vi "FactorPass.vi"(7 "Robot":dbl[](array[numeric]), 8 "error in (no error)":errorcluster, 9 "OffensivePlay":T1=enum."TableWithStriker", 10 "Game":refnum<class "Game.lvclass">, 11 "Utilities in":refnum<class "Utilities.lvclass">) -> (0 "error out":errorcluster, 2 "Critério de marcação Normalizado":dbl, 3 "Utilities out":refnum<class "Utilities.lvclass">)   [LabVIEW 2023, in "Utilities.lvclass"]
uses:
  Utilities.lvclass
  Game_class/Game.lvclass
  Team_class/OffensivePlay.ctl
  Robot_class/roles.ctl
  Game_class/Game.lvclass/Game.ctl
  Object_class/Object.lvclass/Object.ctl
  Referee_class/Referee.lvclass/Referee.ctl
  Team_class/Team.lvclass/Team.ctl
  Robot_class/Robot.lvclass/Robot.ctl
  <vilib>/Analysis/_algsub.llb/Real Vector Norm.vi
  Object_class/Read x.vi
  Object_class/Read y.vi
  Robot_class/Read id.vi
  40316e39-9fcb-4662-8d02-ffa9e406c10e.vi
  Game_class/Read BallRef.vi
  Game_class/Read Referee.vi
  Game_class/Read FieldRef.vi
  Game_class/Read EnemyRef.vi
  Game_class/Read Utilities.lvclass.vi
  Game_class/Read OffensiveTeam.vi
  Team_class/Read RobotRef.vi
  Referee_class/Read enemy_goalie_id.vi
  <vilib>/Array/Sort 2D Array - Pop Stack.vi
  <vilib>/Array/Sort 2D Array - Push Stack.vi
  40316e39-9fcb-4662-8d02-ffa9e406c10e.vi/269d4b3b-47f5-49e3-8884-44851e4dd9d5.vi
  40316e39-9fcb-4662-8d02-ffa9e406c10e.vi/6d99389c-673d-4efb-bf33-19b32bcf4cf8.vi
  Ally_class/Ally.lvclass
  C:/Users/ebert/Documents/codes/SSL/repo/SSL_AI/Team_class/Team.lvclass
  Robot_class/Robot.lvclass
  C:/Users/ebert/Documents/codes/SSL/repo/SSL_AI/Object_class/Object.lvclass
  Enemy_class/Enemy.lvclass
  Ball_class/Ball.lvclass
  Referee_class/Referee.lvclass
  Field_class/Field.lvclass
  <vilib>/Analysis/NI_AALPro.lvlib
panel:
  out "t":dbl
  out "id inimigo \nmaior diferença \nde tempo":dbl
  out "Array out":dbl[][](array[numeric])
  out "Dif. tempo\ninimigo bola":dbl
  out "menor dist":dbl
  out "Robô marcado?":bool=TRUE
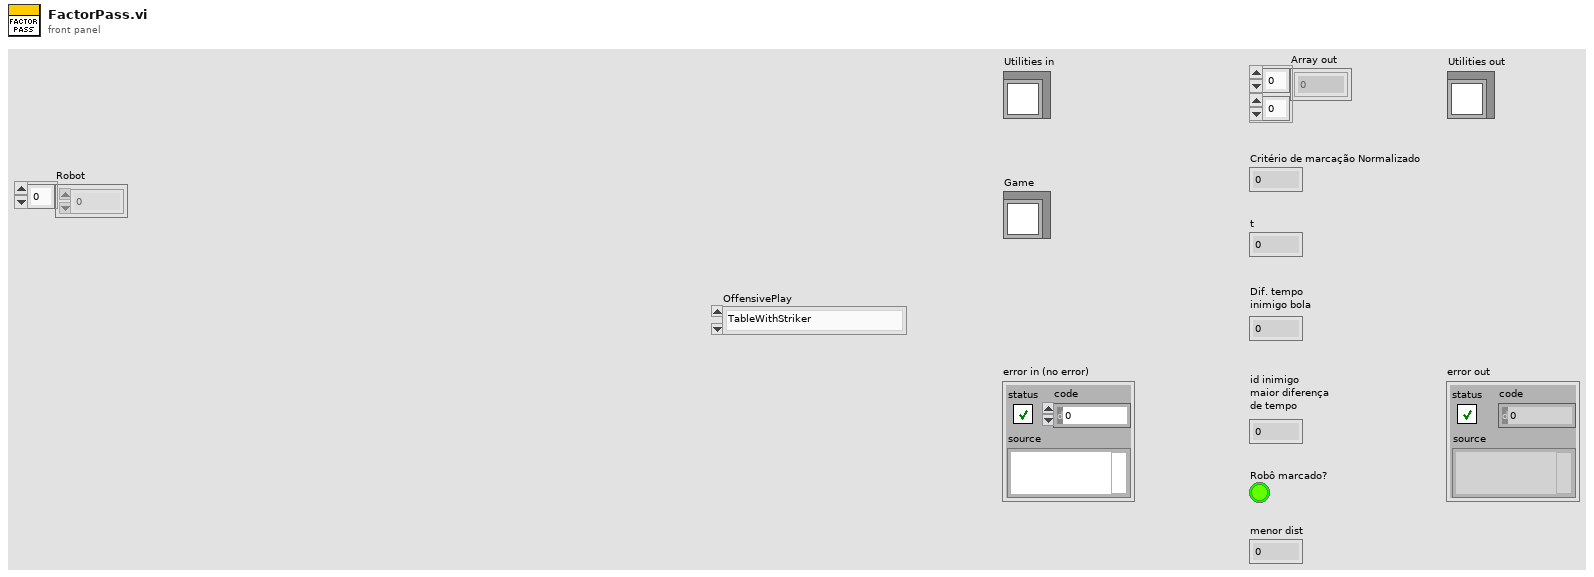
[diagram p1: front panel]
types:
  T1 = typedef "OffensivePlay.ctl" = enum16{"5RobotsPassGamePlay", "5PreparePassGame", "5RobotsKeeperGame", "KeeperPassToStriker", "5RobotsNormalGamePlay", "PrepareKeeperPass", "ACBPass", "ABCPass", "PrepareTriplePass", "TableWithStriker", "TableWith2ndStrikerPlay", "PrepareDoublePass", "PrepareRollToPass", "SimplePass", "PreparePass", "PassToStriker", "BallOutOfField", "PassTo2ndStriker", "StopOffensive", "Prepare Penalty Enemy", "EnemyPossessionAtEnemyField", "EnemyPossesionAtOurField", "TestPlay", "PreparePenaltyAlly", "KickPenaltyAlly", "PrepareKickoffAlly", "PrepareKickoffEnemy", "IndirectEnemy", "DirectEnemy", "PreparePassInGame1", "NormalGame", "DirectKick", "Pass", "Halt", "Timeout", "PassPlay", "PenaltyEnemy"}
  T2 = typedef "roles.ctl" = enum16{"SimpleBallPlacement", "BallPlacementAllyPasser", "BallPlacementAllyReceiver", "BallPlacementEnemy", "5Robots5th", "PassBestReceiver", "5Robots4th", "5Robots3rd", "5Robots2nd", "5Robots1st", "PassBestRobot", "WaitPass", "ABCThirdKicker", "ABCFirstKicker", "ABCSecondKicker", "Tabler", "TableFinalizer", "PrepareRollToPassRoller", "PrepareRollToPassReceiver", "SimplePassRoll", "SimplePassRollReceiver", "PenaltyDefense", "PreparePassReceiver 2", "PreparePassReceiver 1", "PassObserver", "Timeout", "Goto", "ZigZag", "None", "BallOutOfField", "DefenderArea", "Duelist", "AttackerStop", "FollowAttacker", "KeeperRole", "KickPenalty", "AttackerAimGoal", "AttackerBlock", "Marker", "Halt", "Shoot", "PassKicker", "PassReceiver", "TestRole", "PenaltyAttacker"}
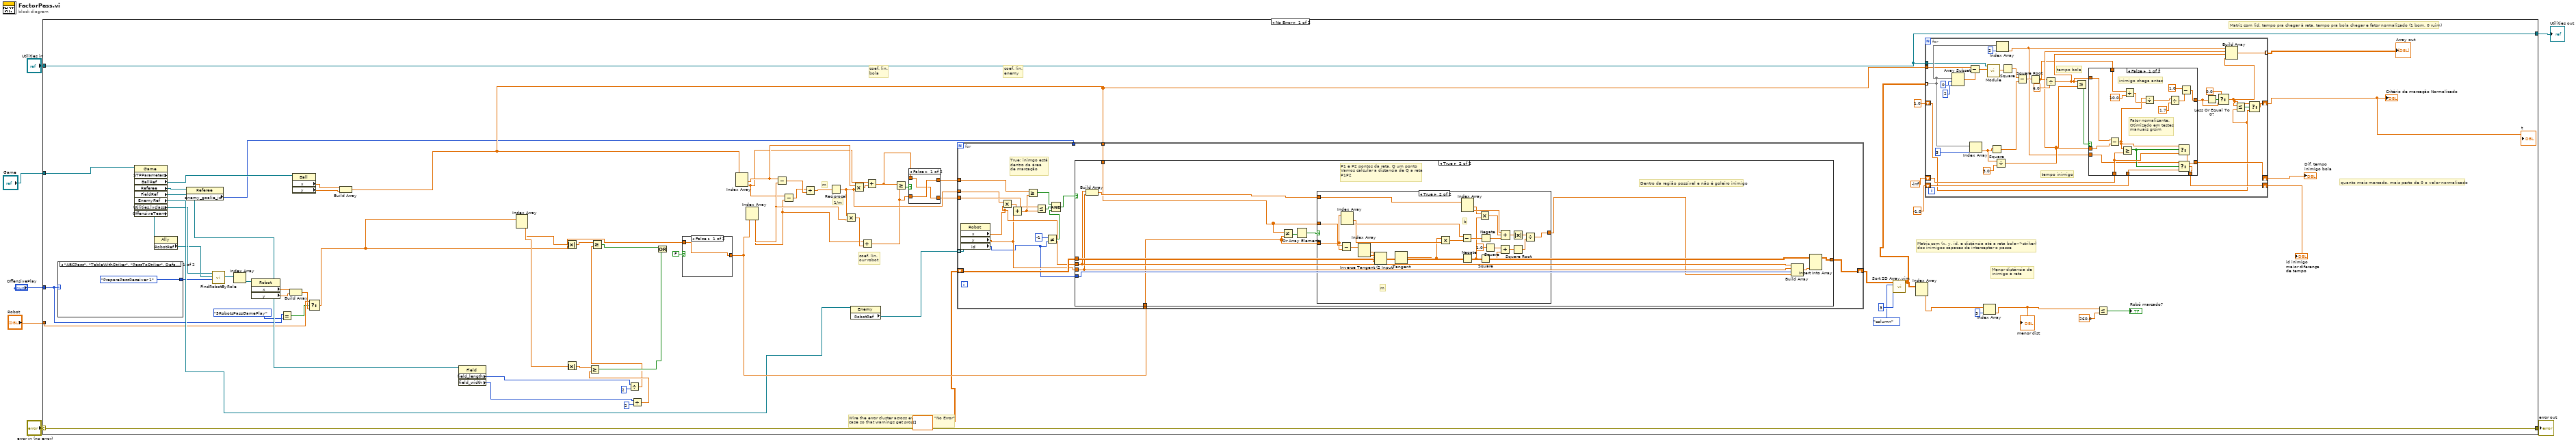
[diagram p0: block diagram]
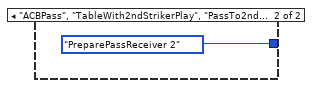
[diagram p2: hidden frame]
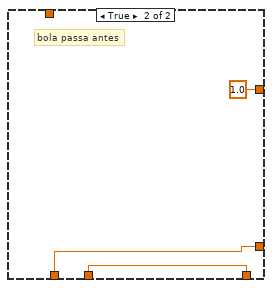
[diagram p3: hidden frame]
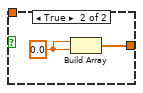
[diagram p4: hidden frame]
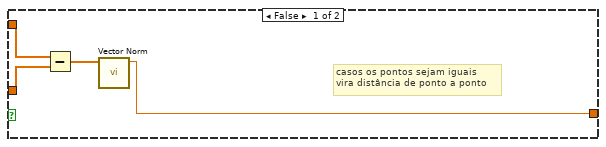
[diagram p7: hidden frame]
diagram:
  n1 = case shown="No Error" "error in (no error)" {
    selector: "error in (no error)" -> [w79 w203]
    tunnel: [w79 w203] -> w6
    tunnel: [w24 w202] -> w4
    tunnel: "Utilities in" -> [w24 w202]
    tunnel: "Game" -> [w23 _]
    tunnel: "OffensivePlay" -> [w10 _]
    tunnel: "Robot" -> [w13 _]
    frame No Error {
      # "Matriz com (id, tempo pra chegar à reta, tempo pra bola chegar e fator normalizado (1 bom, 0 ruim)"
      # "quanto mais marcado, mais perto de 0 o valor normalizado"
      # "Menor distância de \ninimigo à reta"
      # "Matriz com (x, y, id, e distância até a reta bola-->striker) \ndos inimigos capazes de interceptar o passe"
      # "coef. lin.\nbola"
      # "coef. lin.\nenemy"
      # "coef. lin.\nour robot"
      # "1/m"
      # "m"
      # "Wire the error cluster across even in the \"No Error\"\ncase so that warnings get propagated."
      n2 = case shown="\"ABCPass\", \"TableWithStriker\", \"PassToStriker\", Default" w10 {
        tunnel: [roles."PreparePassReceiver 1" ("role") roles."PreparePassReceiver 2" ("role")] -> w22
        frame "ABCPass", "TableWithStriker", "PassToStriker", Default {
        }
        frame "ACBPass", "TableWith2ndStrikerPlay", "PassTo2ndStriker" {
        }
      }
      n3 = property class="Game" props=["STPParameters", "BallRef", "Referee", "FieldRef", "EnemyRef", "Utilities.lvclass", "OffensiveTeam"](reference=w23) -> ("BallRef"=w35:refnum<class "Ball.lvclass">, "Referee"=w31:refnum<class "Referee.lvclass">, "FieldRef"=w29:refnum<class "Field.lvclass">, "EnemyRef"=w26:refnum<class "Enemy.lvclass">, "Utilities.lvclass"=w21:refnum<class "Utilities.lvclass">, "OffensiveTeam"=w16:refnum<class "Ally.lvclass">)  [unwired: 1 in, 3 out]
      n4 = property class="Ally"(reference=w16) -> ("RobotRef"=w15:refnum<class "Robot.lvclass">[])  [unwired: 1 in, 2 out]
      n5 = property class="Referee"(reference=w31) -> ("enemy_goalie_id"=w30:i32)  [unwired: 1 in, 2 out]
      n6 = call "FindRobotByRole.vi"("role"=w22, "RobotRef"=w15, "Utilities in"=w21) -> ("Robots"=w20:refnum<class "Robot.lvclass">[])  [unwired: 6 in, 2 out]
      n7 = Index Array(array=w20) -> (element=w19:refnum<class "Robot.lvclass">)  [unwired: 1 in]
      n8 = property class="Robot"(reference=w19) -> ("x"=w18:dbl, "y"=w17:dbl)  [unwired: 1 in, 2 out]
      n9 = Equal?(x=w10, y=OffensivePlay."5RobotsPassGamePlay") -> (x = y?=w11:bool)
      n10 = Build Array(w18, w17) -> (w12:dbl[])
      n11 = property class="Ball"(reference=w35) -> ("x"=w34:dbl, "y"=w33:dbl)  [unwired: 1 in, 2 out]
      n12 = Select(t=w13, s=w11, f=w12) -> (s? t:f=w14:dbl[])
      n13 = Build Array(w34, w33) -> (w32:dbl[])
      n14 = property class="Field"(reference=w29) -> ("field_length"=w28:i32, "field_width"=w27:i32)  [unwired: 1 in, 2 out]
      n15 = Index Array(array=w14) -> (element #1=w74:dbl, element #2=w75:dbl)  [unwired: 2 in]
      n16 = Absolute Value(x=w74) -> (abs(x)=w55:dbl)
      n17 = Absolute Value(x=w75) -> (abs(x)=w57:dbl)
      n18 = Divide(x=w28, y=2) -> (x/y=w56:dbl)
      n19 = Greater Or Equal?(x=w55, y=w56) -> (x >= y?=w59:bool)
      n20 = Divide(x=w27, y=u32 2) -> (x/y=w58:dbl)
      n21 = Greater Or Equal?(x=w57, y=w58) -> (x >= y?=w60:bool)
      n22 = Or(x=w59, y=w60) -> ()  [unwired: 1 out]
      n23 = case shown="False" FALSE {
        tunnel: [w135 w136] -> w61
        tunnel: w14 -> [w135 _]
        frame False {
        }
        frame True {
          w137 = 0.0
          n24 = Build Array(w137, w137) -> (w136:dbl[])
        }
      }
      n25 = Index Array(array=w32) -> (element #1=w71:dbl, element #2=w37:dbl)  [unwired: 2 in]
      n26 = Index Array(array=w61) -> (element #1=w70:dbl, element #2=w38:dbl)  [unwired: 2 in]
      n27 = Subtract(x=w71, y=w70) -> (x-y=w40:dbl)
      n28 = Subtract(x=w37, y=w38) -> (x-y=w39:dbl)
      n29 = Divide(x=w39, y=w40) -> (x/y=w36:dbl)
      n30 = Reciprocal(x=w36) -> (1/x=w73:dbl)
      n31 = Multiply(x=w73, y=w70) -> (x*y=w69:dbl)
      n32 = property class="Enemy"(reference=w26) -> ("RobotRef"=w25:refnum<class "Robot.lvclass">[])  [unwired: 1 in, 2 out]
      n33 = Multiply(x=w71, y=w73) -> (x*y=w72:dbl)
      n34 = Add(x=w38, y=w69) -> (x+y=w43:dbl)
      n35 = Add(x=w37, y=w72) -> (x+y=w42:dbl)
      n36 = Greater Or Equal?(x=w42, y=w43) -> (x >= y?=w41:bool)
      n37 = case shown="False" w41 {
        tunnel: [w139 w141] -> w44
        tunnel: w42 -> [w138 w141]
        tunnel: [w138 w140] -> w45
        tunnel: w43 -> [w139 w140]
        frame False {
        }
        frame True {
        }
      }
      n38 = for {
        tunnel: w73 -> [w149]
        shift-right: [w158] -> w48
        shift-left: dbl[][] [] -> [w159]
        tunnel: w44 -> [w153]
        tunnel: w45 -> [w152]
        tunnel: w32 -> [w151]
        tunnel: w61 -> [w150]
        tunnel: w30 -> [_]
        tunnel: w25 -> [w146] mode=indexing
        # "True: inimgo está \ndentro da área\nde marcação"
        n39 = property class="Robot"(reference=w146) -> ("x"=w145:dbl, "y"=w144:dbl, "id"=w143:i32)  [unwired: 1 in, 2 out]
        n40 = Multiply(x=w149, y=w145) -> (x*y=w148:dbl)
        n41 = Add(x=w148, y=w144) -> (x+y=w157:dbl)
        n42 = Greater Or Equal?(x=w153, y=w157) -> (x >= y?=w155:bool)
        n43 = Less Or Equal?(x=w152, y=w157) -> (x <= y?=w156:bool)
        n44 = Not Equal?(x=-1, y=w143) -> (x != y?=w147:bool)
        n45 = Compound Arithmetic op=AND(w155, w156, w147) -> (w154:bool)
        n46 = case shown="True" w154 {
          tunnel: w159 -> [w160 w172]
          tunnel: [w160 w171] -> w158
          tunnel: w145 -> [_ w168]
          tunnel: w144 -> [_ w167]
          tunnel: w143 -> [_ w170]
          tunnel: w151 -> [_ w163]
          tunnel: w150 -> [_ w162]
          frame False {
            # "Fora da região possível ou é goleiro inimigo"
          }
          frame True {
            # "P1 e P2 pontos da reta, Q um ponto\nVamos calcular a distancia de Q a reta \nP1P2"
            # "Dentro da região possível e não é goleiro inimigo"
            n47 = Build Array(w168, w167) -> (w164:dbl[])
            n48 = Not Equal?(x=w163, y=w162) -> (x != y?=w166:bool[])
            n49 = Or Array Elements(Boolean array=w166) -> (logical OR=w165:bool)
            n50 = case shown="True" w165 {
              tunnel: w163 -> [w175 w201]
              tunnel: w162 -> [_ w197]
              tunnel: w164 -> [w176 w193]
              tunnel: [w173 w179] -> w161
              frame False {
                # "casos os pontos sejam iguais\nvira distância de ponto a ponto"
                n51 = Subtract(x=w176, y=w175) -> (x-y=w174:dbl[])
                n52 = call-poly <vilib>:"Vector Norm.vi"("Input Vector"=w174) -> ("norm"=w173:dbl)  [unwired: 9 in, 1 out]
              }
              frame True {
                # "b"
                # "m"
                n53 = Subtract(x=w201, y=w197) -> (x-y=w200:dbl[])
                n54 = Index Array(array=w197) -> (element #1=w195:dbl, element #2=w196:dbl)  [unwired: 2 in]
                n55 = Index Array(array=w200) -> (element #1=w198:dbl, element #2=w199:dbl)  [unwired: 2 in]
                n56 = Inverse Tangent (2 Input)(1:w198, 2:w199) -> (0:w178:dbl)
                n57 = Tangent(1:w178) -> (0:w177:dbl)
                n58 = Multiply(x=w177, y=w195) -> (x*y=w194:dbl)
                n59 = Subtract(x=w196, y=w194) -> (x-y=w189:dbl)
                n60 = Index Array(array=w193) -> (element #1=w191:dbl, element #2=w192:dbl)  [unwired: 2 in]
                n61 = Negate(x=w177) -> (-x=w185:dbl)
                n62 = Multiply(x=w191, y=w185) -> (x*y=w190:dbl)
                n63 = Square(x=w185) -> (x^2=w183:dbl)
                n64 = Negate(x=w189) -> (-x=w188:dbl)
                n65 = Square(x=1.0) -> (x^2=w184:dbl)
                n66 = Add(x=w184, y=w183) -> (x+y=w182:dbl)
                n67 = Compound Arithmetic op=ADD(w192, w190, w188) -> (w187:dbl)
                n68 = Absolute Value(x=w187) -> (abs(x)=w181:dbl)
                n69 = Square Root(x=w182) -> (sqrt(x)=w180:dbl)
                n70 = Divide(x=w181, y=w180) -> (x/y=w179:dbl)
              }
            }
            n71 = Build Array(w168, w167, w170, w161) -> (w169:dbl[])
            n72 = Insert Into Array(array=w172, new element=w169) -> (w171:dbl[][])  [unwired: 2 in]
          }
        }
      }
      n73 = call "Sort 2D Array.vim"("index"=3, "dimension to index (column)"=enum16{"column", "row"}."column", "2D array"=w48) -> ("sorted 2D array"=w64:dbl[][])  [unwired: 7 in, 1 out]
      n74 = Index Array(array=w64) -> (element=w63:dbl[])  [unwired: 2 in]
      n75 = for {
        tunnel: w32 -> [w86]
        tunnel: w64 -> [w99] mode=indexing
        shift-right: [w95] -> w76
        shift-left: -inf -> [w104]
        tunnel: [w103] -> w66 mode=indexing
        shift-right: [w98] -> w68
        shift-left: -1.0 ("Numeric") -> [w96]
        shift-right: [w90] -> w77
        shift-left: 1.0 ("t") -> [w82]
        tunnel: w24 -> [w84]
        # "tempo inimigo"
        # "tempo bola"
        n76 = Array Subset(array=w99, index=0, length=2) -> (w87:dbl[])
        n77 = Subtract(x=w86, y=w87) -> (x-y=w85:dbl[])
        n78 = Index Array(array=w99, index=3) -> (element=w107:dbl)
        n79 = call "Module.vi"("2D vector"=w85, "Utilities in"=w84) -> ("Modulo"=w83:dbl)  [unwired: 7 in, 2 out]
        n80 = Square(x=w107) -> (x^2=w110:dbl)
        n81 = Divide(x=w107, y=3.0) -> (x/y=w101:dbl)
        n82 = Index Array(array=w99, index=2) -> (element=w97:dbl)
        n83 = Square(x=w83) -> (x^2=w111:dbl)
        n84 = Subtract(x=w111, y=w110) -> (x-y=w109:dbl)
        n85 = Square Root(x=w109) -> (sqrt(x)=w94:dbl)
        n86 = Divide(x=w94, y=6.0) -> (x/y=w102:dbl)
        n87 = Less Or Equal?(x=w102, y=w101) -> (x <= y?=w105:bool)
        n88 = case shown="False" w105 {
          tunnel: w101 -> [w129 _]
          tunnel: w102 -> [w130 _]
          tunnel: [w121 w134] -> w95
          tunnel: w104 -> [w131 w134]
          tunnel: [w127 w133] -> w98
          tunnel: w97 -> [w126 _]
          tunnel: w96 -> [w125 w133]
          tunnel: w94 -> [w124 _]
          tunnel: [w116 1.0] -> w92
          frame False {
            # "Fator nomalizante.\nOtimizado em testes\nmanuais grsim"
            # "inimigo chega antes"
            n89 = Subtract(x=w130, y=w129) -> (x-y=w115:dbl)
            n90 = Greater Or Equal?(x=w115, y=w131) -> (x >= y?=w128:bool)
            n91 = Divide(x=w124, y=10.0) -> (x/y=w122:dbl)
            n92 = Divide(x=w115, y=w122) -> (x/y=w120:dbl)
            n93 = Divide(x=w120, y=1.7) -> (x/y=w117:dbl)
            n94 = Select(t=w115, s=w128, f=w131) -> (s? t:f=w121:dbl)
            n95 = Select(t=w126, s=w128, f=w125) -> (s? t:f=w127:dbl)
            n96 = Subtract(x=1.0, y=w117) -> (x-y=w116:dbl)
          }
          frame True {
            # "bola passa antes"
          }
        }
        n97 = Less Or Equal To 0?(x=w92) -> (x <= 0?=w93:bool)
        n98 = Select(t=0.0, s=w93, f=w92) -> (s? t:f=w89:dbl)
        n99 = Build Array(w97, w101, w102, w89) -> (w103:dbl[])
        n100 = Less Or Equal?(x=w89, y=w82) -> (x <= y?=w88:bool)
        n101 = Select(t=w89, s=w88, f=w82) -> (s? t:f=w90:dbl)
      }
      "Dif. tempo\ninimigo bola" <- w76
      "Array out" <- w66
      "id inimigo \nmaior diferença \nde tempo" <- w68
      "Critério de marcação Normalizado" <- w77
      "t" <- w77
      n102 = Index Array(array=w63, index=3) -> (element=w62:dbl)
      "menor dist" <- w62
      n103 = Less Or Equal?(x=w62, y=260.0) -> (x <= y?=→"Robô marcado?":bool)
    }
    frame Error {
    }
  }
  "error out" <- w6
  "Utilities out" <- w4
